vi "fit - 1 over T.vi"(10 "what points":dbl[](array[numeric]), 11 "temperature points":dbl[](array[numeric])) -> (0 "best fit parameters":dbl[](array[numeric]), 2 "what points out":dbl[](array[numeric]), 3 "temperature points out":dbl[](array[numeric]), 4 "covariance":T1, 5 "residue":dbl)   [LabVIEW 2014]
uses:
  <vilib>/Analysis/Matrix/Datatypes/RealMatrix.ctl
  <vilib>/gmath/NumericalOptimization/LM model function reference.ctl
  <vilib>/gmath/NumericalOptimization/Nonlinear Curve Fit LM.vi
  <vilib>/gmath/NI_Gmath.lvlib
  <vilib>/Analysis/Matrix/NI_Matrix.lvlib
panel:
  in  "power":dbl
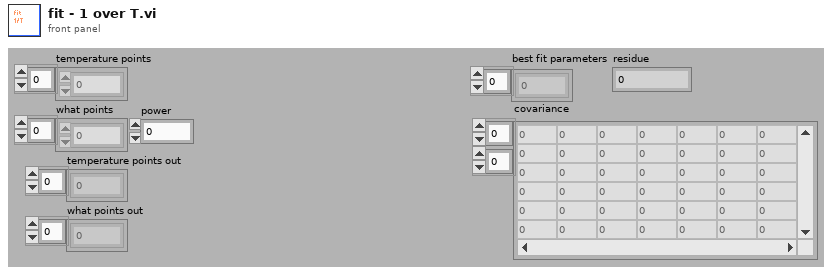
[diagram p1: front panel]
types:
  T1 = typedef "NI_Matrix.lvlib/RealMatrix.ctl" = dbl[][]
  T2 = typedef "NI_Gmath.lvlib/LM model function reference.ctl" = refnum<vi>
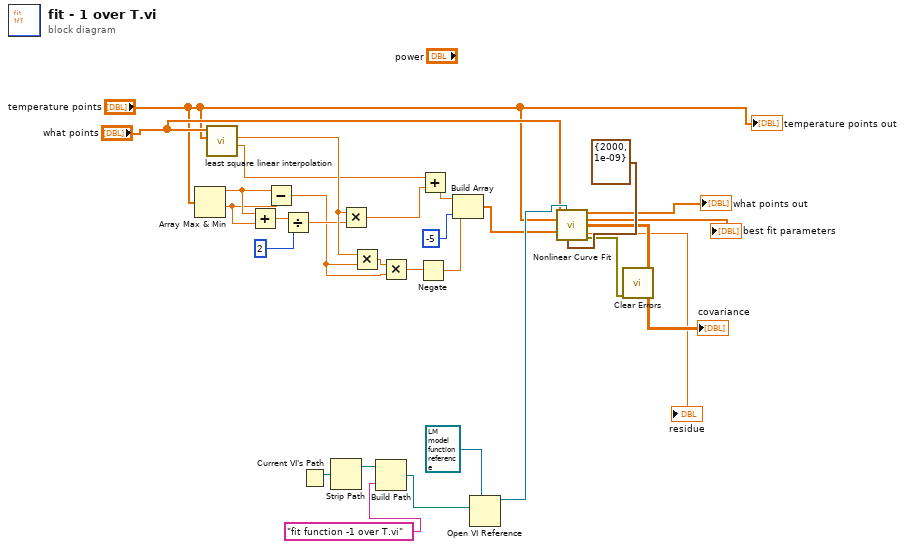
[diagram p0: block diagram]
diagram:
  n1 = Array Max & Min(array="temperature points") -> (max value=w27:dbl, min value=w26:dbl)  [unwired: 2 out]
  n2 = call "least square linear interpolation.vi"("X"="temperature points", "Y"="what points") -> ("intercept"=w20:dbl, "slope"=w23:dbl)  [unwired: 8 in]
  n3 = Add(x=w27, y=w26) -> (x+y=w25:dbl)
  n4 = Subtract(x=w27, y=w26) -> (x-y=w18:dbl)
  n5 = Divide(x=w25, y=2) -> (x/y=w22:dbl)
  n6 = Current VI's Path() -> (path=w15:path)
  n7 = Strip Path(path=w15) -> (stripped path=w16:path)  [unwired: 1 out]
  n8 = Multiply(x=w23, y=w22) -> (x*y=w21:dbl)
  n9 = Multiply(x=w23, y=w18) -> (x*y=w17:dbl)
  n10 = Build Path(base path=w16, name or relative path="fit function -1 over T.vi" ("f(x,a) VI name Complex")) -> (appended path=w13:path)
  n11 = Multiply(x=w17, y=w18) -> (x*y=w5:dbl)
  n12 = Negate(x=w5) -> (-x=w4:dbl)
  n13 = Add(x=w20, y=w21) -> (x+y=w19:dbl)
  n14 = Build Array(w19, w4, -5) -> (w6:dbl[])
  n15 = Open VI Reference(type specifier VI Refnum (for type only)=T2 refnum ("f(x,a)"), vi path=w13) -> (vi reference=w11:T2)  [unwired: 1 in, 4 out]
  n16 = call-poly <vilib>:"Nonlinear Curve Fit.vi"("Y"="what points", "f(x,a)"=w11, "X"="temperature points", "initial parameters"=w6, "termination"=cluster{"max iteration":i32, "tolerance":dbl} {"max iteration"=2000, "tolerance"=1e-09}) -> ("best nonlinear fit"=→"what points out":dbl[], "best fit parameters"=→"best fit parameters":dbl[], "covariance"=→"covariance":T1, "residue"=→"residue":dbl, "error out"=w28:errorcluster)  [unwired: 5 in, 1 out]
  n17 = call <vilib>:"Clear Errors.vi"("error in (no error)"=w28) -> ()  [unwired: 5 in, 2 out]
  "temperature points out" <- "temperature points"
